vi "Get Status Channels.vi"(8 "error in (no error)":errorcluster, 11 "VeriStand Data Sharing Framework in":refnum<class "VeriStand DSF.lvclass">) -> (0 "error out":errorcluster, 3 "VeriStand Data Sharing Framework out":refnum<class "VeriStand DSF.lvclass">)   [LabVIEW 2017, in "DSF Engine.lvlib" / "VeriStand DSF.lvclass"]
uses:
  VeriStand DSF.lvclass
  VeriStand DSF.lvclass/VeriStand DSF.ctl
  <vilib>/NI Veristand/Custom Device API/Data Access Type.ctl
  DSF Core.lvlibp/Typedefs/DSF Data Type.ctl
  DSF Core.lvlibp/Classes/Buffer/Buffer.lvclass
  <vilib>/NI Veristand/Custom Device API/Custom Device API.lvlib
  Shared/DSF Shared.lvlib
  DSF Core.lvlibp/Classes/Framework/Framework.lvclass
  DSF Core.lvlibp
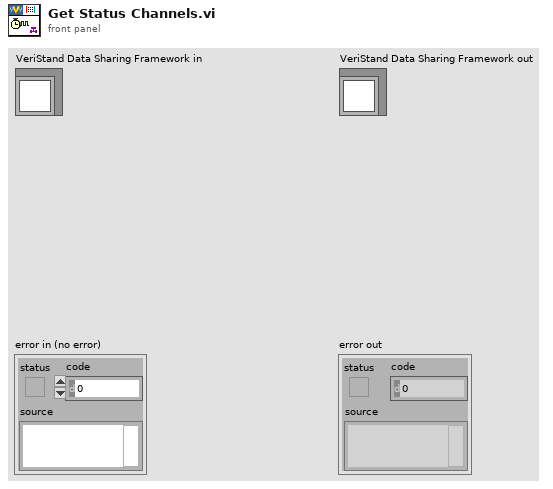
[diagram p1: front panel]
types:
  T1 = typedef "Custom Device API.lvlib/Custom Device Item Ref.ctl" = u64
  T2 = typedef "Custom Device API.lvlib/Data Access Type.ctl" = enum16{"Read", "Write"}
  T3 = typedef "DSF Core.lvlibp/DSF Data Type.ctl" = enum8{"Bool", "SGL", "DBL", "I8", "I16", "I32", "I64", "U8", "U16", "U32", "U64"}
  T4 = typedef "Custom Device API.lvlib/Data Reference.ctl" = i32
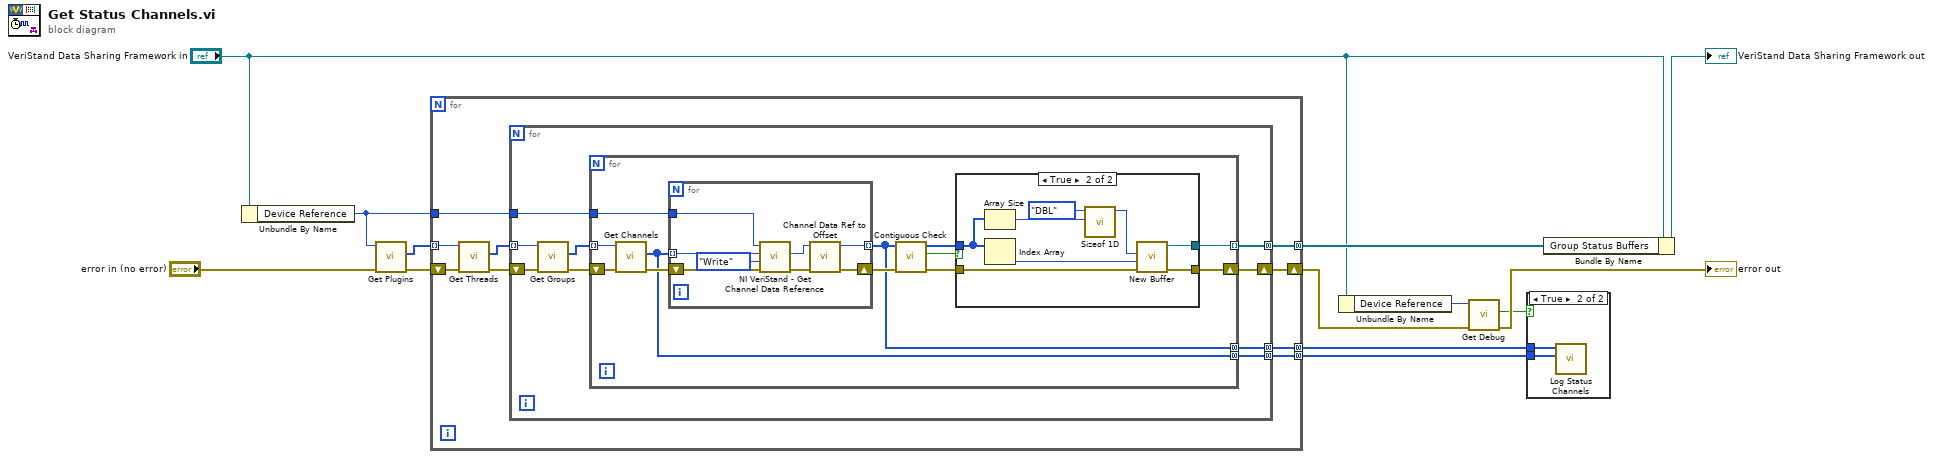
[diagram p0: block diagram]
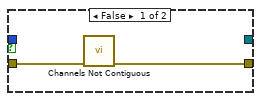
[diagram p2: hidden frame]
diagram:
  n1 = Unbundle By Name("VeriStand Data Sharing Framework in") -> ("Device Reference"=w8:T1)
  n2 = call "Get Plugins.vi"("error in (no error)"="error in (no error)", "Item Ref in"=w8) -> ("error out"=w13:errorcluster, "Plugin refs"=w12:T1[])  [unwired: 7 in, 1 out]
  n3 = for {
    tunnel: w12 -> [w19] mode=indexing
    tunnel: w8 -> [w21]
    shift-right: [w22] -> w6
    shift-left: w13 -> [w20]
    tunnel: [w16] -> w10 mode=concatenating
    tunnel: [w15] -> w4 mode=concatenating
    tunnel: [w14] -> w3 mode=concatenating
    n4 = call "Get Threads.vi"("error in (no error)"=w20, "Item Ref in"=w19) -> ("error out"=w18:errorcluster, "Plugin refs"=w17:T1[])  [unwired: 7 in, 1 out]
    n5 = for {
      tunnel: w17 -> [w28] mode=indexing
      tunnel: w21 -> [w31]
      shift-right: [w30] -> w22
      shift-left: w18 -> [w29]
      tunnel: [w25] -> w16 mode=concatenating
      tunnel: [w24] -> w15 mode=concatenating
      tunnel: [w23] -> w14 mode=concatenating
      n6 = call "Get Groups.vi"("error in (no error)"=w29, "Plugin Ref in"=w28) -> ("error out"=w27:errorcluster, "Group refs"=w26:T1[])  [unwired: 7 in, 1 out]
      n7 = for {
        tunnel: w26 -> [w42] mode=indexing
        tunnel: w31 -> [w40]
        shift-right: [w35] -> w30
        shift-left: w27 -> [w43]
        tunnel: [w34] -> w25 mode=indexing
        tunnel: [w33] -> w24 mode=concatenating
        tunnel: [w32] -> w23 mode=concatenating
        n8 = call "Get Channels.vi"("error in (no error)"=w43, "Item Ref in"=w42) -> ("error out"=w41:errorcluster, "Channels refs"=w33:T1[])  [unwired: 7 in, 1 out]
        n9 = for {
          shift-right: [w50] -> w39
          shift-left: w41 -> [w49]
          tunnel: [w47] -> w32 mode=indexing
          tunnel: w40 -> [w45]
          tunnel: w33 -> [w44] mode=indexing
          n10 = call <vilib>:"NI VeriStand - Get Channel Data Reference.vi"("error in (no error)"=w49, "Access"=Data_Access_Type."Write", "Channel Ref in"=w44, "Device Ref in"=w45) -> ("error out"=w51:errorcluster, "Channel Data Reference"=w48:T4)  [unwired: 5 in, 1 out]
          n11 = call "Channel Data Ref to Offset.vi"("error in (no error)"=w51, "Channel Data Reference"=w48) -> ("error out"=w50:errorcluster, "channel offset"=w47:u64)  [unwired: 8 in]
        }
        n12 = call "Contiguous Check.vi"("error in (no error)"=w39, "channel offsets in"=w32) -> ("error out"=w38:errorcluster, "contiguous?"=w37:bool, "channel offsets out"=w36:u64[])  [unwired: 7 in]
        n13 = case shown="True" w37 {
          tunnel: w38 -> [w53 w61]
          tunnel: w36 -> [_ w57]
          tunnel: [w52 w54] -> w35
          tunnel: [_ w55] -> w34
          frame False {
            n14 = call "Channels Not Contiguous.vi"("error in (no error)"=w53) -> ("error out"=w52:errorcluster)  [unwired: 10 in]
          }
          frame True {
            n15 = Array Size(array=w57) -> (size(s)=w60:i32)
            n16 = Index Array(array=w57) -> (element=w58:u64)  [unwired: 1 in]
            n17 = call "Sizeof 1D.vi"("count"=w60, "data type"=DSF_Data_Type."DBL") -> ("size in bytes"=w56:u64)  [unwired: 9 in]
            n18 = call "New Buffer.vi"("error in (no error)"=w61, "buffer offset (0)"=w58, "buffer size"=w56) -> ("error out"=w54:errorcluster, "Buffer out"=w55:refnum<class "Buffer.lvclass">)  [unwired: 7 in]
          }
        }
      }
    }
  }
  n19 = Unbundle By Name("VeriStand Data Sharing Framework in") -> ("Device Reference"=w7:T1)
  n20 = call "Get Debug.vi"("error in (no error)"=w6, "Item Ref in"=w7) -> ("error out"=→"error out":errorcluster, "debug"=w1:bool)  [unwired: 7 in, 1 out]
  n21 = case shown="True" w1 {
    tunnel: w4 -> [_ w63]
    tunnel: w3 -> [_ w62]
    frame False {
    }
    frame True {
      n22 = call "Log Status Channels.vi"("status channels refs"=w63, "status channel offsets"=w62) -> ()  [unwired: 10 in]
    }
  }
  n23 = Bundle By Name(cluster="VeriStand Data Sharing Framework in", "Group Status Buffers"=w10) -> (→"VeriStand Data Sharing Framework out":refnum<class "VeriStand DSF.lvclass">)
